vi "EnergyStorage_Write Control.vi"(10 "EnergyStorage_Control":cluster{"kW setpoint":dbl}, 11 "EnergyStorage in":refnum<class "EnergyStorage.lvclass">) -> (3 "EnergyStorage out":refnum<class "EnergyStorage.lvclass">)   [LabVIEW 2015, in "EnergyStorage.lvclass"]
uses:
  EnergyStorage.lvclass
  EnergyStorage.lvclass/EnergyStorage.ctl
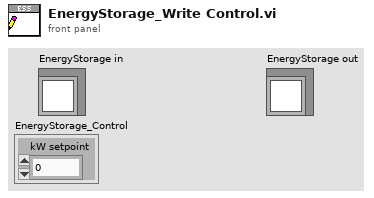
[diagram p1: front panel]
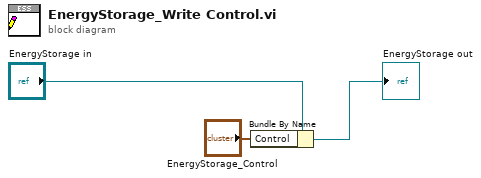
[diagram p0: block diagram]
diagram:
  n1 = Bundle By Name(cluster="EnergyStorage in", "Control"="EnergyStorage_Control") -> (→"EnergyStorage out":refnum<class "EnergyStorage.lvclass">)
